vi "Library.vi"(0 "Message_command_in":T1, 3 "error in (no error)":errorcluster) -> (7 "Message_command out":T1, 10 "error out":errorcluster)   [LabVIEW 2025]
uses:
  Command_Message.ctl
  <vilib>/Utility/error.llb/Trim Whitespace One-Sided.vi
panel:
  out "result string":string
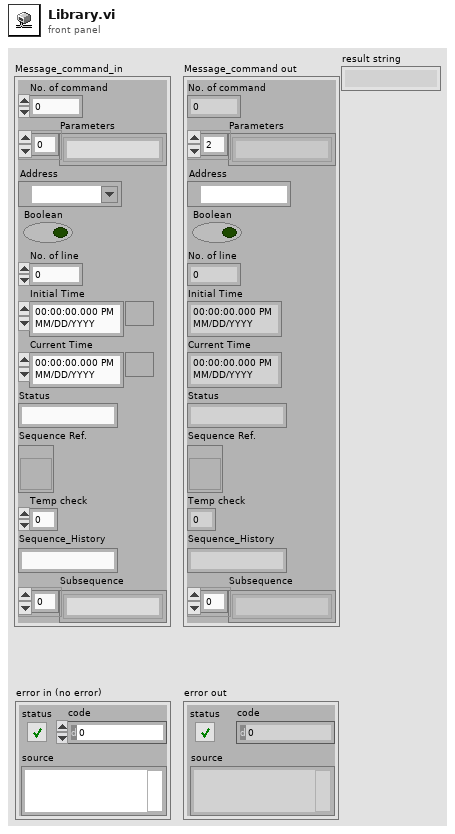
[diagram p1: front panel]
types:
  T1 = typedef "Command_Message.ctl" = cluster{"No. of command":i32, "Parameters":string[], "Address":refnum<visa-resource-name>, "Boolean":bool, "No. of line":i32, "Initial Time":timestamp, "Current Time":timestamp, "Status":string, "Sequence Ref.":refnum<vi>, "Temp check":i32, "Sequence_History":string, "Subsequence":string[]}
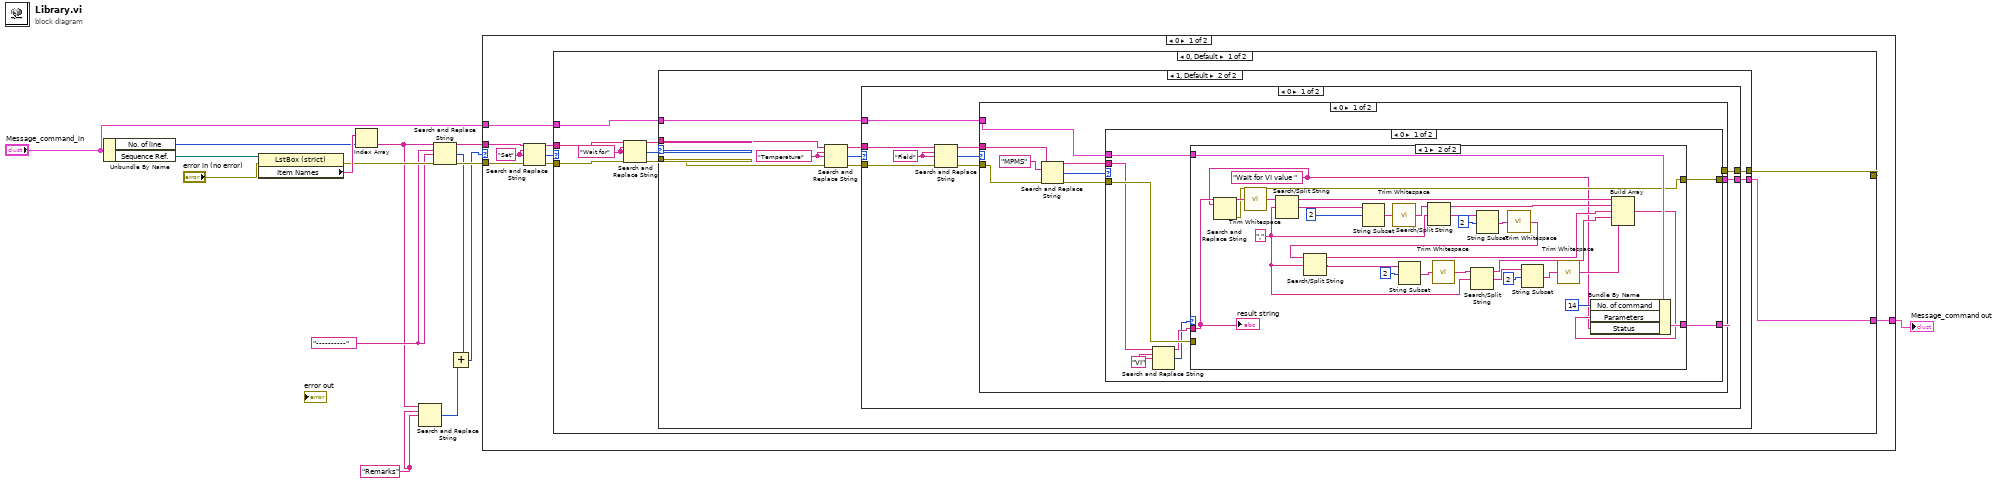
[diagram p0: block diagram]
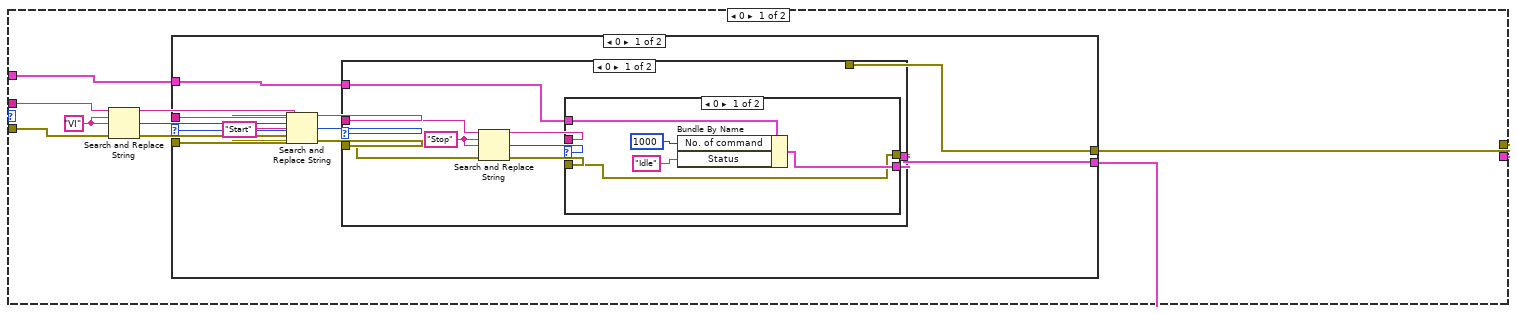
[diagram p2: hidden frame]
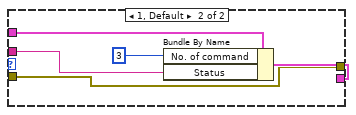
[diagram p3: hidden frame]
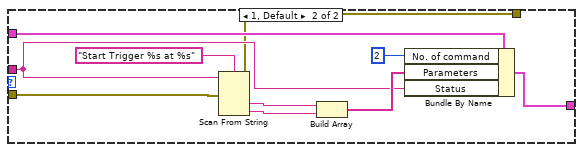
[diagram p4: hidden frame]
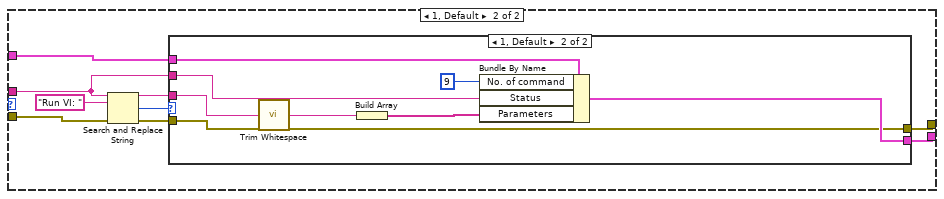
[diagram p5: hidden frame]
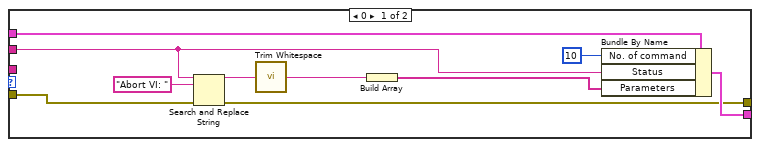
[diagram p6: hidden frame]
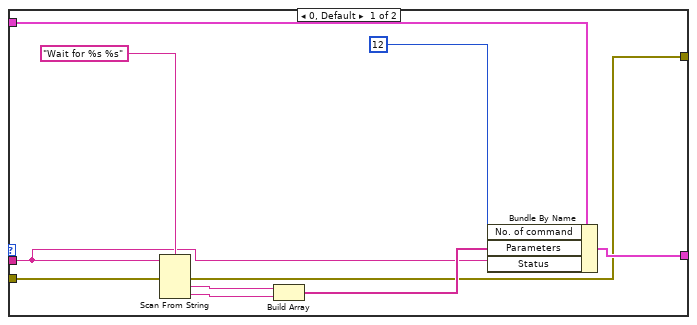
[diagram p7: hidden frame]
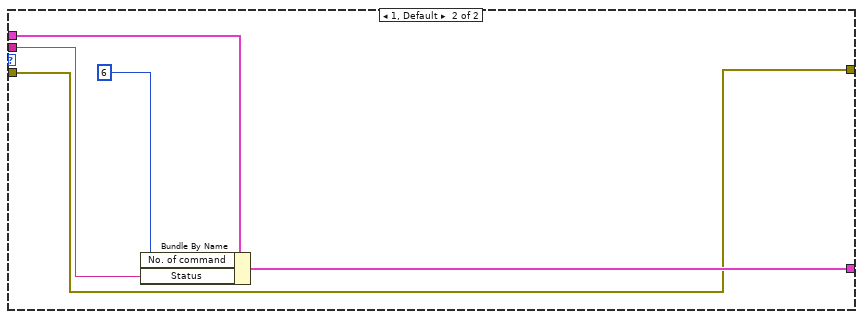
[diagram p8: hidden frame]
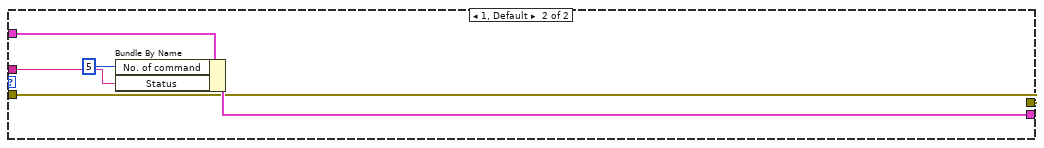
[diagram p9: hidden frame]
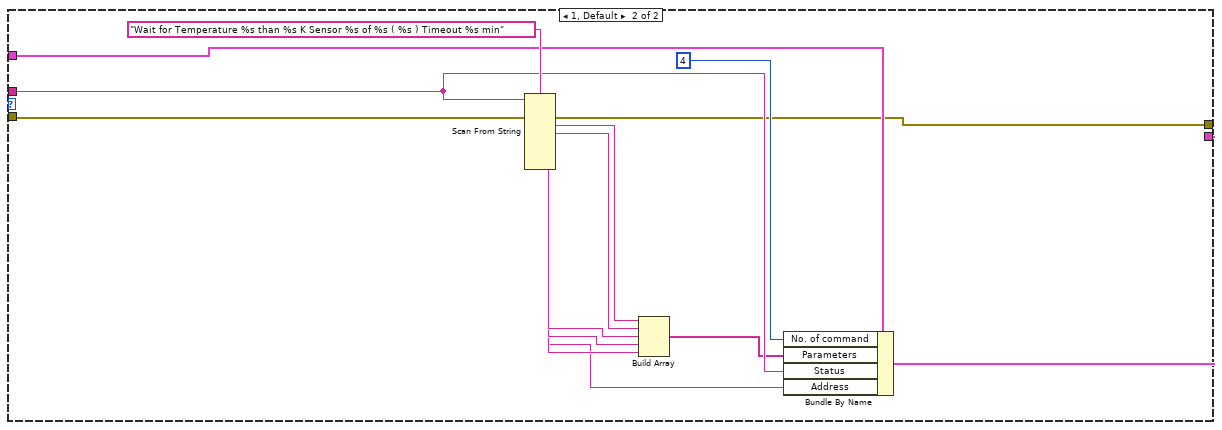
[diagram p10: hidden frame]
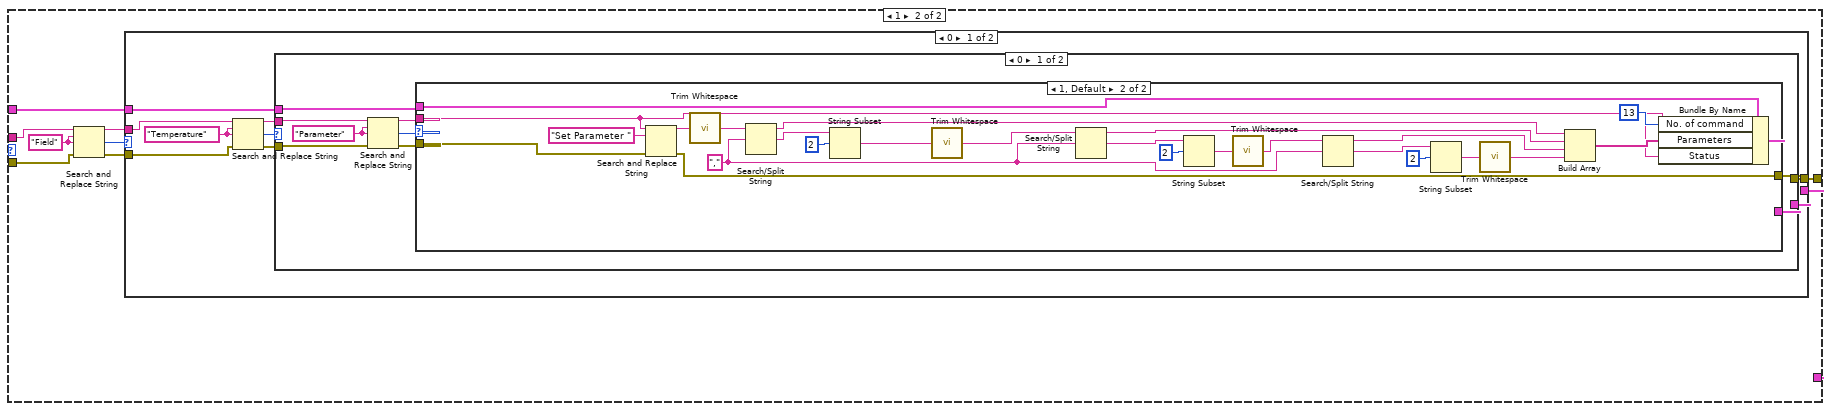
[diagram p11: hidden frame]
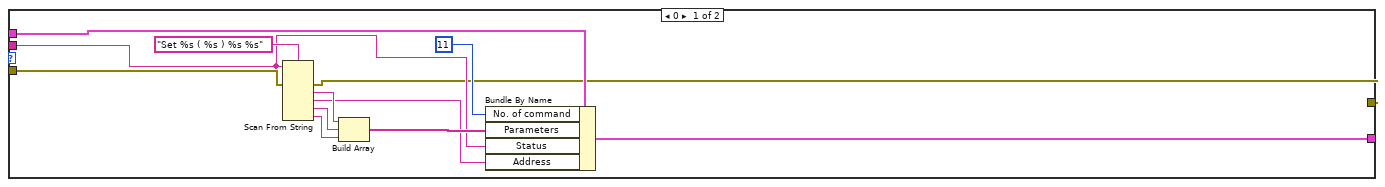
[diagram p12: hidden frame]
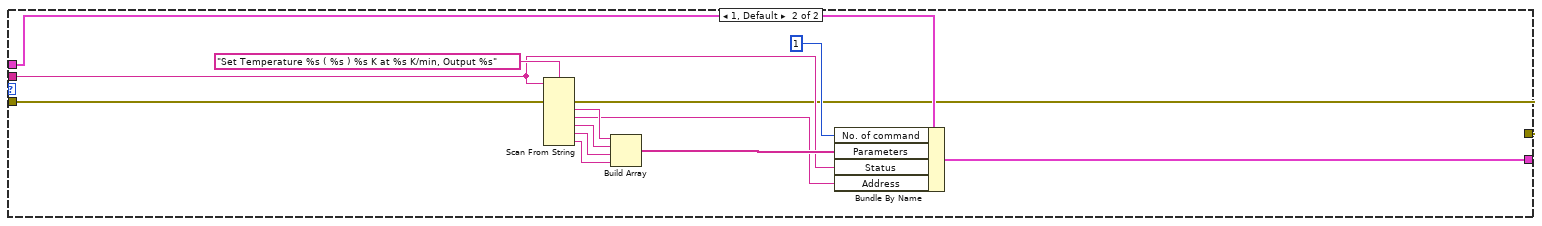
[diagram p13: hidden frame]
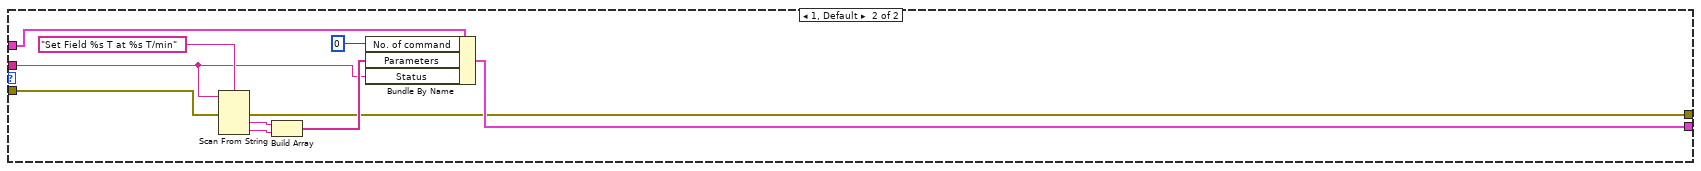
[diagram p14: hidden frame]
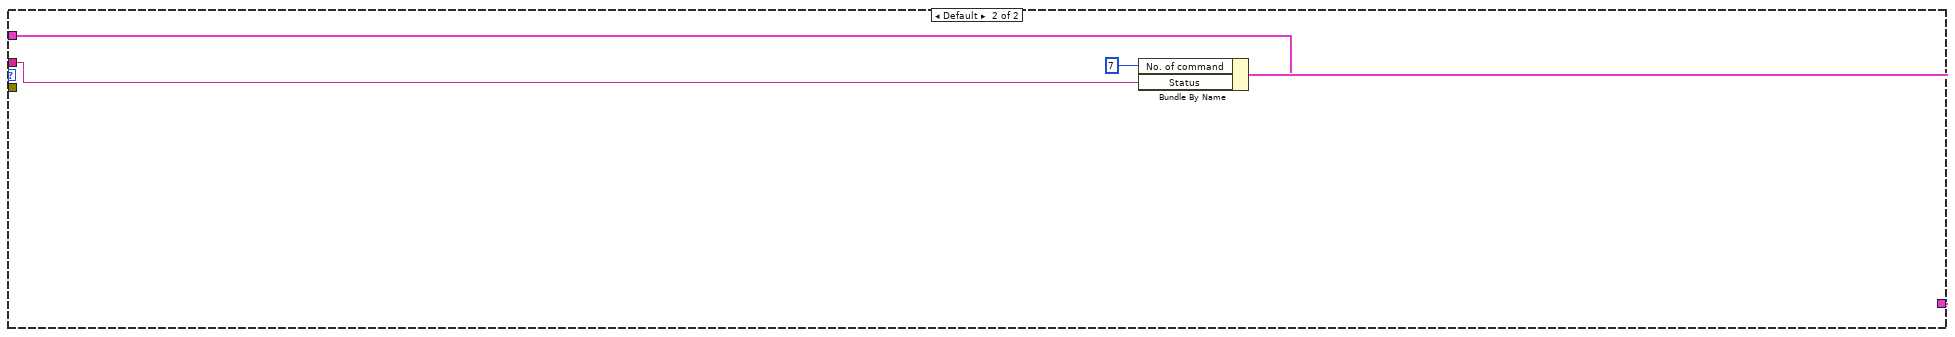
[diagram p15: hidden frame]
diagram:
  w5 = "Remarks" ("search string")
  w6 = "----------" ("search string")
  n1 = Unbundle By Name("Message_command_in") -> ("No. of line"=w12:i32, "Sequence Ref."=w13:refnum<vi>)
  n2 = property on="Property Node" class="LstBox (strict)"(reference=w13, error in="error in (no error)") -> (error out=w8:errorcluster, "Item Names"=w15:string[])  [unwired: 1 out]
  n3 = Index Array(array=w15, index=w12) -> (element=w2:string)
  n4 = Search and Replace String(input string=w2, search string=w5, replace string=w5) -> (number of replacements=w3:i32)  [unwired: 5 in, 3 out]
  n5 = Search and Replace String(input string=w2, search string=w6, replace string=w6, error in=w8) -> (result string=w9:string, number of replacements=w4:i32, error out=w7:errorcluster)  [unwired: 4 in, 1 out]
  n6 = Add(x=w4, y=w3) -> (x+y=w1:i32)
  n7 = case shown="0" w1 {
    tunnel: w7 -> [w23 _]
    tunnel: "Message_command_in" -> [w18 w294]
    tunnel: [w17 w295] -> w10
    tunnel: w9 -> [w16 w297]
    frame 0 {
      w22 = "Set" ("search string")
      n8 = Search and Replace String(input string=w16, search string=w22, replace string=w22, error in=w23) -> (result string=w20:string, number of replacements=w21:i32, error out=w19:errorcluster)  [unwired: 4 in, 1 out]
      n9 = case shown="0, Default" w21 {
        tunnel: w20 -> [w32 w214]
        tunnel: w19 -> [w30 w213]
        tunnel: w18 -> [w26 w208]
        tunnel: [w25 w207] -> w17
        tunnel: [w24 w206] -> _
        frame 0, Default {
          w31 = "Wait for" ("search string")
          n10 = Search and Replace String(input string=w32, search string=w31, replace string=w31, error in=w30) -> (result string=w28:string, number of replacements=w29:i32, error out=w27:errorcluster)  [unwired: 4 in, 1 out]
          n11 = case shown="1, Default" w29 {
            tunnel: w28 -> [w41 w115]
            tunnel: w27 -> [w39 w113]
            tunnel: w26 -> [w35 w110]
            tunnel: [w34 w108] -> w25
            tunnel: [w33 w107] -> w24
            frame 0 {
              w40 = "VI" ("search string")
              n12 = Search and Replace String(input string=w41, search string=w40, replace string=w40, error in=w39) -> (result string=w37:string, number of replacements=w38:i32, error out=w36:errorcluster)  [unwired: 4 in, 1 out]
              n13 = case shown="0" w38 {
                tunnel: w37 -> [w50 w84]
                tunnel: w36 -> [w49 w87]
                tunnel: w35 -> [w45 w83]
                tunnel: [w44 w82] -> w34
                tunnel: [w43 w80] -> w33
                frame 0 {
                  w48 = "Start" ("search string")
                  n14 = Search and Replace String(input string=w50, search string=w48, replace string=w48, error in=w49) -> (result string=w47:string, number of replacements=w42:i32, error out=w46:errorcluster)  [unwired: 4 in, 1 out]
                  n15 = case shown="0" w42 {
                    tunnel: w47 -> [w57 w74]
                    tunnel: w46 -> [w51 w78]
                    tunnel: w45 -> [w59 w72]
                    tunnel: [w58 w71] -> w44
                    tunnel: [w52 w70] -> w43
                    frame 0 {
                      w56 = "Stop" ("input string")
                      n16 = Search and Replace String(input string=w57, search string=w56, replace string=w56, error in=w51) -> (result string=w54:string, number of replacements=w55:i32, error out=w53:errorcluster)  [unwired: 4 in, 1 out]
                      n17 = case shown="0" w55 {
                        tunnel: w59 -> [w63 w68]
                        tunnel: [w64 w67] -> w58
                        tunnel: w54 -> [_ w66]
                        tunnel: w53 -> [w60 w65]
                        tunnel: [w60 w65] -> w52
                        frame 0 {
                          n18 = Bundle By Name(cluster=w63, "No. of command"=1000, "Status"="Idle") -> (w64:T1)
                        }
                        frame 1, Default {
                          n19 = Bundle By Name(cluster=w68, "No. of command"=3, "Status"=w66) -> (w67:T1)
                        }
                      }
                    }
                    frame 1, Default {
                      n20 = Scan From String(format string="Start Trigger %s at %s", input string=w74, error in=w78) -> (error out=w70:errorcluster, output 1=w77:string, output 2=w76:string)  [unwired: 3 in, 2 out]
                      n21 = Build Array(w77, w76) -> (w75:string[])
                      n22 = Bundle By Name(cluster=w72, "No. of command"=2, "Parameters"=w75, "Status"=w74) -> (w71:T1)
                    }
                  }
                }
                frame 1, Default {
                  n23 = Search and Replace String(input string=w84, search string="Run VI: ", error in=w87) -> (result string=w85:string, number of replacements=w86:i32, error out=w81:errorcluster)  [unwired: 5 in, 1 out]
                  n24 = case shown="1, Default" w86 {
                    tunnel: w85 -> [_ w106]
                    tunnel: w84 -> [w94 w102]
                    tunnel: w83 -> [w92 w101]
                    tunnel: [w91 w100] -> w82
                    tunnel: w81 -> [w90 w99]
                    tunnel: [w89 w99] -> w80
                    frame 0 {
                      n25 = Search and Replace String(input string=w94, search string="Abort VI: " ("format string"), error in=w90) -> (result string=w97:string, error out=w89:errorcluster)  [unwired: 5 in, 2 out]
                      n26 = call <vilib>:"Trim Whitespace.vi"("string"=w97) -> ("trimmed string"=w96:string)  [unwired: 1 in]
                      n27 = Build Array(w96) -> (w95:string[])
                      n28 = Bundle By Name(cluster=w92, "No. of command"=10, "Status"=w94, "Parameters"=w95) -> (w91:T1)
                    }
                    frame 1, Default {
                      n29 = call <vilib>:"Trim Whitespace.vi"("string"=w106) -> ("trimmed string"=w105:string)  [unwired: 1 in]
                      n30 = Build Array(w105) -> (w103:string[])
                      n31 = Bundle By Name(cluster=w101, "No. of command"=9, "Status"=w102, "Parameters"=w103) -> (w100:T1)
                    }
                  }
                }
              }
            }
            frame 1, Default {
              w114 = "Temperature" ("search string")
              n32 = Search and Replace String(input string=w115, search string=w114, replace string=w114, error in=w113) -> (result string=w111:string, number of replacements=w112:i32, error out=w109:errorcluster)  [unwired: 4 in, 1 out]
              n33 = case shown="0" w112 {
                tunnel: w111 -> [w124 w195]
                tunnel: w110 -> [w120 w203]
                tunnel: w109 -> [w123 w193]
                tunnel: [w119 w202] -> w108
                tunnel: [w116 w192] -> w107
                frame 0 {
                  w122 = "Field" ("search string")
                  n34 = Search and Replace String(input string=w124, search string=w122, replace string=w122, error in=w123) -> (result string=w118:string, number of replacements=w121:i32, error out=w117:errorcluster)  [unwired: 4 in, 1 out]
                  n35 = case shown="0" w121 {
                    tunnel: w118 -> [w133 w188]
                    tunnel: w120 -> [w127 w191]
                    tunnel: [w128 w190] -> w119
                    tunnel: w117 -> [w131 w187]
                    tunnel: [w125 w187] -> w116
                    frame 0 {
                      n36 = Search and Replace String(input string=w133, search string="MPMS", error in=w131) -> (result string=w129:string, number of replacements=w130:i32, error out=w126:errorcluster)  [unwired: 5 in, 1 out]
                      n37 = case shown="0" w130 {
                        tunnel: w129 -> [w137 w185]
                        tunnel: [w139 w184] -> w128
                        tunnel: w127 -> [w140 w183]
                        tunnel: w126 -> [w141 w182]
                        tunnel: [w138 w182] -> w125
                        frame 0 {
                          w134 = "VI" ("search string")
                          n38 = Search and Replace String(input string=w137, search string=w134, replace string=w134) -> (result string=w136:string, number of replacements=w135:i32)  [unwired: 5 in, 2 out]
                          n39 = case shown="1" w135 {
                            tunnel: w141 -> [w150 _]
                            tunnel: w140 -> [w147 w181]
                            tunnel: [w146 w180] -> w139
                            tunnel: w136 -> [w142 w154]
                            tunnel: [w143 w155] -> w138
                            frame 0, Default {
                              n40 = Scan From String(format string="Wait for %s %s", input string=w142, error in=w150) -> (error out=w143:errorcluster, output 1=w149:string, output 2=w148:string)  [unwired: 3 in, 2 out]
                              n41 = Build Array(w149, w148) -> (w144:string[])
                              n42 = Bundle By Name(cluster=w147, "No. of command"=12, "Parameters"=w144, "Status"=w142) -> (w146:T1)
                            }
                            frame 1 {
                              w172 = "," ("search string/char (-)")
                              w152 = "Wait for VI value " ("search string")
                              n43 = Search and Replace String(input string=w154, search string=w152) -> (result string=w159:string, error out=w155:errorcluster)  [unwired: 6 in, 2 out]
                              n44 = call <vilib>:"Trim Whitespace.vi"("string"=w159) -> ("trimmed string"=w160:string)  [unwired: 1 in]
                              n45 = Search/Split String(string=w160, search string/char (-)=w172) -> (substring before match=w175:string, match + rest of string=w162:string)  [unwired: 1 in, 1 out]
                              n46 = String Subset(string=w162, offset (0)=2) -> (substring=w163:string)  [unwired: 1 in]
                              n47 = call <vilib>:"Trim Whitespace.vi"("string"=w163) -> ("trimmed string"=w157:string)  [unwired: 1 in]
                              n48 = Search/Split String(string=w157, search string/char (-)=w172) -> (substring before match=w176:string, match + rest of string=w165:string)  [unwired: 1 in, 1 out]
                              n49 = String Subset(string=w165, offset (0)=2) -> (substring=w166:string)  [unwired: 1 in]
                              n50 = call <vilib>:"Trim Whitespace.vi"("string"=w166) -> ("trimmed string"=w158:string)  [unwired: 1 in]
                              n51 = Search/Split String(string=w158, search string/char (-)=w172) -> (substring before match=w177:string, match + rest of string=w171:string)  [unwired: 1 in, 1 out]
                              n52 = String Subset(string=w171, offset (0)=2) -> (substring=w170:string)  [unwired: 1 in]
                              n53 = call <vilib>:"Trim Whitespace.vi"("string"=w170) -> ("trimmed string"=w173:string)  [unwired: 1 in]
                              n54 = Search/Split String(string=w173, search string/char (-)=w172) -> (substring before match=w178:string, match + rest of string=w174:string)  [unwired: 1 in, 1 out]
                              n55 = String Subset(string=w174, offset (0)=2) -> (substring=w168:string)  [unwired: 1 in]
                              n56 = call <vilib>:"Trim Whitespace.vi"("string"=w168) -> ("trimmed string"=w153:string)  [unwired: 1 in]
                              n57 = Build Array(w175, w176, w177, w178, w153) -> (w156:string[])
                              n58 = Bundle By Name(cluster=w181, "No. of command"=14, "Parameters"=w156, "Status"=w152) -> (w180:T1)
                              "result string" <- w154
                            }
                          }
                        }
                        frame 1, Default {
                          n59 = Bundle By Name(cluster=w183, "No. of command"=6, "Status"=w185) -> (w184:T1)
                        }
                      }
                    }
                    frame 1, Default {
                      n60 = Bundle By Name(cluster=w191, "No. of command"=5, "Status"=w188) -> (w190:T1)
                    }
                  }
                }
                frame 1, Default {
                  n61 = Scan From String(format string="Wait for Temperature %s than %s K Sensor %s of %s ( %s ) Timeout %s min", input string=w195, error in=w193) -> (error out=w192:errorcluster, output 1=w201:string, output 2=w200:string, output 3=w199:string, output 4=w198:string, output 5=w196:string, output 6=w197:string)  [unwired: 7 in, 2 out]
                  n62 = Build Array(w201, w200, w199, w198, w197) -> (w194:string[])
                  n63 = Bundle By Name(cluster=w203, "No. of command"=4, "Parameters"=w194, "Status"=w195, "Address"=w196) -> (w202:T1)
                }
              }
            }
          }
        }
        frame 1 {
          w212 = "Field" ("search string")
          n64 = Search and Replace String(input string=w214, search string=w212, replace string=w212, error in=w213) -> (result string=w210:string, number of replacements=w211:i32, error out=w209:errorcluster)  [unwired: 4 in, 1 out]
          n65 = case shown="0" w211 {
            tunnel: w210 -> [w223 w287]
            tunnel: w209 -> [w222 w292]
            tunnel: w208 -> [w217 w286]
            tunnel: [w216 w285] -> w207
            tunnel: [w215 w284] -> w206
            frame 0 {
              w221 = "Temperature" ("search string")
              n66 = Search and Replace String(input string=w223, search string=w221, replace string=w221, error in=w222) -> (result string=w219:string, number of replacements=w220:i32, error out=w218:errorcluster)  [unwired: 4 in, 1 out]
              n67 = case shown="0" w220 {
                tunnel: w219 -> [w232 w273]
                tunnel: w218 -> [w231 w282]
                tunnel: w217 -> [w226 w277]
                tunnel: [w225 w276] -> w216
                tunnel: [w224 w271] -> w215
                frame 0 {
                  w230 = "Parameter" ("search string")
                  n68 = Search and Replace String(input string=w232, search string=w230, replace string=w230, error in=w231) -> (result string=w227:string, number of replacements=w229:i32, error out=w228:errorcluster)  [unwired: 4 in, 1 out]
                  n69 = case shown="1, Default" w229 {
                    tunnel: w228 -> [w243 w264]
                    tunnel: w227 -> [w237 w266]
                    tunnel: w226 -> [w235 w268]
                    tunnel: [w234 w267] -> w225
                    tunnel: [w233 w256] -> w224
                    frame 0 {
                      n70 = Scan From String(format string="Set %s ( %s ) %s %s", input string=w237, error in=w243) -> (error out=w233:errorcluster, output 1=w242:string, output 2=w236:string, output 3=w241:string, output 4=w240:string)  [unwired: 5 in, 2 out]
                      n71 = Build Array(w242, w241, w240) -> (w239:string[])
                      n72 = Bundle By Name(cluster=w235, "No. of command"=11, "Parameters"=w239, "Status"=w237, "Address"=w236) -> (w234:T1)
                    }
                    frame 1, Default {
                      w259 = "," ("search string/char (-)")
                      n73 = Search and Replace String(input string=w266, search string="Set Parameter ", error in=w264) -> (result string=w255:string, error out=w256:errorcluster)  [unwired: 5 in, 2 out]
                      n74 = call <vilib>:"Trim Whitespace.vi"("string"=w255) -> ("trimmed string"=w254:string)  [unwired: 1 in]
                      n75 = Search/Split String(string=w254, search string/char (-)=w259) -> (substring before match=w263:string, match + rest of string=w252:string)  [unwired: 1 in, 1 out]
                      n76 = String Subset(string=w252, offset (0)=2) -> (substring=w251:string)  [unwired: 1 in]
                      n77 = call <vilib>:"Trim Whitespace.vi"("string"=w251) -> ("trimmed string"=w262:string)  [unwired: 1 in]
                      n78 = Search/Split String(string=w262, search string/char (-)=w259) -> (substring before match=w261:string, match + rest of string=w249:string)  [unwired: 1 in, 1 out]
                      n79 = String Subset(string=w249, offset (0)=2) -> (substring=w248:string)  [unwired: 1 in]
                      n80 = call <vilib>:"Trim Whitespace.vi"("string"=w248) -> ("trimmed string"=w260:string)  [unwired: 1 in]
                      n81 = Search/Split String(string=w260, search string/char (-)=w259) -> (substring before match=w258:string, match + rest of string=w246:string)  [unwired: 1 in, 1 out]
                      n82 = String Subset(string=w246, offset (0)=2) -> (substring=w245:string)  [unwired: 1 in]
                      n83 = call <vilib>:"Trim Whitespace.vi"("string"=w245) -> ("trimmed string"=w257:string)  [unwired: 1 in]
                      n84 = Build Array(w263, w261, w258, w257) -> (w270:string[])
                      n85 = Bundle By Name(cluster=w268, "No. of command"=13, "Parameters"=w270, "Status"=w266) -> (w267:T1)
                    }
                  }
                }
                frame 1, Default {
                  n86 = Scan From String(format string="Set Temperature %s ( %s ) %s K at %s K/min, Output %s", input string=w273, error in=w282) -> (error out=w271:errorcluster, output 1=w281:string, output 2=w272:string, output 3=w280:string, output 4=w279:string, output 5=w278:string)  [unwired: 6 in, 2 out]
                  n87 = Build Array(w281, w280, w279, w278) -> (w274:string[])
                  n88 = Bundle By Name(cluster=w277, "No. of command"=1, "Parameters"=w274, "Status"=w273, "Address"=w272) -> (w276:T1)
                }
              }
            }
            frame 1, Default {
              n89 = Scan From String(format string="Set Field %s T at %s T/min", input string=w287, error in=w292) -> (error out=w284:errorcluster, output 1=w291:string, output 2=w290:string)  [unwired: 3 in, 2 out]
              n90 = Build Array(w291, w290) -> (w288:string[])
              n91 = Bundle By Name(cluster=w286, "No. of command"=0, "Parameters"=w288, "Status"=w287) -> (w285:T1)
            }
          }
        }
      }
    }
    frame Default {
      n92 = Bundle By Name(cluster=w294, "No. of command"=7, "Status"=w297) -> (w295:T1)
    }
  }
  "Message_command out" <- w10
